vi "Main template.vi"() -> ()   [LabVIEW 2016]
panel:
  out "Finger 5 (little)":dbl(knob) scale=0.0..180.0
  out "Finger 3 (middle)":dbl(knob) scale=0.0..180.0
  out "Finger 4 (ring)":dbl(knob) scale=0.0..180.0
  out "Finger 2 (index)":dbl(knob) scale=0.0..180.0
  out "Finger 1 (thumb)":dbl(knob) scale=0.0..180.0
  out "Finger 5 (individual)":bool
  out "Finger 4 (individual)":bool
  out "Finger 3 (individual)":bool
  out "Finger 2 (individual)":bool
  out "Finger 1 (individual)":bool
  in  "Finger 5 (individual)":bool
  in  "FInger 4 (individual)":bool
  in  "Finger 3 (individual)":bool
  in  "Finger 2 (individual)":bool
  in  "Finger 1 (individual)":bool
  in  "stop":bool
  out "Test 4":bool
  out "Test 3":bool
  out "Test 2":bool
  out "Test 1":bool
  in  "Boolean 2":bool
  in  "Boolean 1":bool
  # "Joakim Nylander Nordström\ncomp3\nNeurotechnology"
  # "Booleans representing the first two\nbits in message from comp2"
  # "Gauge (mätare) displaying\neach finger angle"
  # "Booleans for the last five bits\ncontrolling individual fingers"
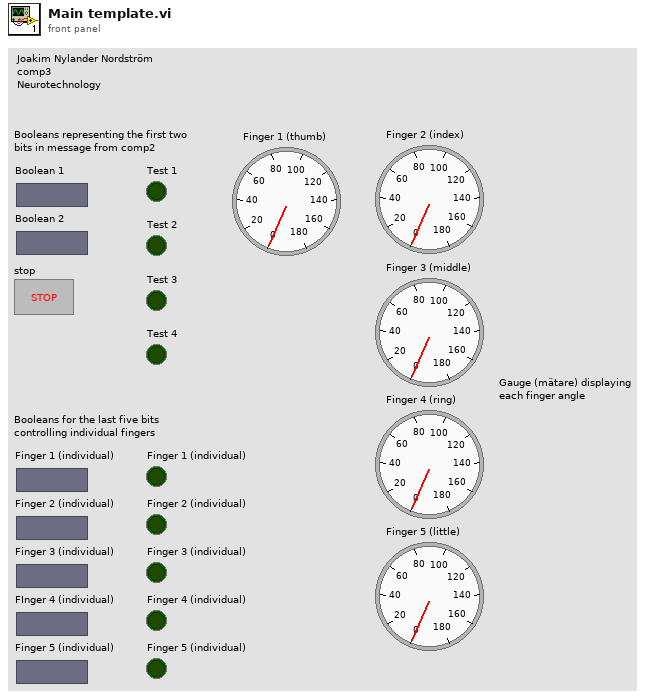
[diagram p1: front panel]
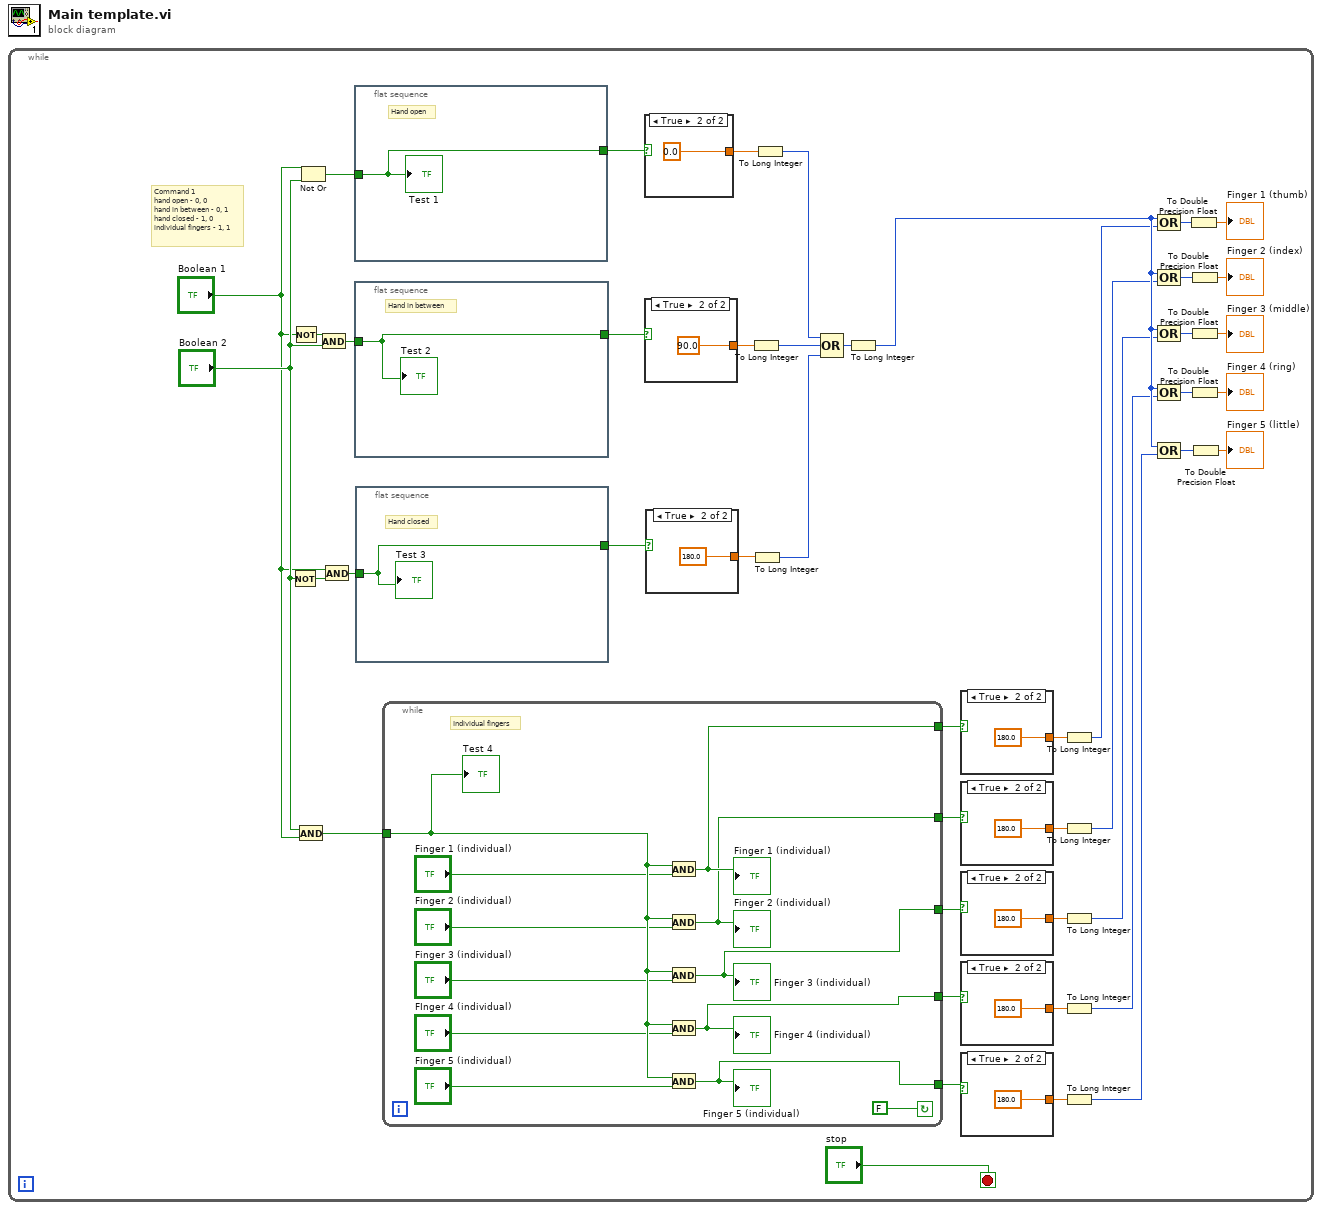
[diagram p0: block diagram]
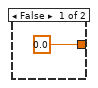
[diagram p2: hidden frame]
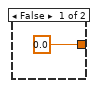
[diagram p3: hidden frame]
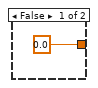
[diagram p4: hidden frame]
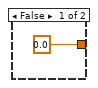
[diagram p5: hidden frame]
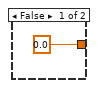
[diagram p6: hidden frame]
diagram:
  n1 = while {
    stop <- "stop" stop-if-true
    # "Command 1\nhand open - 0, 0\nhand in between - 0, 1\nhand closed - 1, 0\nindividual fingers - 1, 1"
    n2 = Not(x="Boolean 2") -> (.not. x?=w44:bool)
    n3 = Not(x="Boolean 1") -> (.not. x?=w45:bool)
    n4 = And(x="Boolean 2", y="Boolean 1") -> (x .and. y?=w43:bool)
    n5 = Not Or(1:"Boolean 2", 2:"Boolean 1") -> (0:w42:bool)
    n6 = And(x=w45, y="Boolean 2") -> (x .and. y?=w41:bool)
    n7 = And(x="Boolean 1", y=w44) -> (x .and. y?=w39:bool)
    n8 = flat-sequence {
      tunnel: w42 -> [w61]
      tunnel: [w61] -> w36
      frame #0 {
        # "Hand open"
        "Test 1" <- w61
      }
    }
    n9 = flat-sequence {
      tunnel: w41 -> [w60]
      tunnel: [w60] -> w38
      frame #0 {
        # "Hand in between"
        "Test 2" <- w60
      }
    }
    n10 = flat-sequence {
      tunnel: w39 -> [w59]
      tunnel: [w59] -> w34
      frame #0 {
        # "Hand closed"
        "Test 3" <- w59
      }
    }
    n11 = while {
      tunnel: w43 -> [w73]
      tunnel: [w66] -> w17
      tunnel: [w65] -> w16
      tunnel: [w64] -> w15
      tunnel: [w63] -> w14
      tunnel: [w62] -> w13
      stop <- FALSE continue-if-true
      # "Individual fingers"
      n12 = And(x=w73, y="Finger 1 (individual)") -> (x .and. y?=w66:bool)
      "Finger 1 (individual)" <- w66
      n13 = And(x=w73, y="Finger 2 (individual)") -> (x .and. y?=w65:bool)
      "Finger 2 (individual)" <- w65
      n14 = And(x=w73, y="Finger 3 (individual)") -> (x .and. y?=w64:bool)
      "Finger 3 (individual)" <- w64
      n15 = And(x=w73, y="FInger 4 (individual)") -> (x .and. y?=w63:bool)
      "Finger 4 (individual)" <- w63
      n16 = And(x=w73, y="Finger 5 (individual)") -> (x .and. y?=w62:bool)
      "Finger 5 (individual)" <- w62
      "Test 4" <- w73
    }
    n17 = case shown="True" w36 {
      tunnel: [_ 0.0] -> w35
      frame False {
      }
      frame True {
      }
    }
    n18 = case shown="True" w38 {
      tunnel: [_ 90.0] -> w37
      frame False {
      }
      frame True {
      }
    }
    n19 = case shown="True" w34 {
      tunnel: [_ 180.0] -> w31
      frame False {
      }
      frame True {
      }
    }
    n20 = To Long Integer(number=w37) -> (32bit integer=w32:i32)
    n21 = To Long Integer(number=w31) -> (32bit integer=w30:i32)
    n22 = To Long Integer(number=w35) -> (32bit integer=w33:i32)
    n23 = Compound Arithmetic op=OR(w33, w32, w30) -> (w29:i32)
    n24 = To Long Integer(number=w29) -> (32bit integer=w28:i32)
    n25 = case shown="True" w17 {
      tunnel: [0.0 180.0] -> w12
      frame False {
      }
      frame True {
      }
    }
    n26 = case shown="True" w16 {
      tunnel: [0.0 180.0] -> w11
      frame False {
      }
      frame True {
      }
    }
    n27 = case shown="True" w15 {
      tunnel: [0.0 180.0] -> w10
      frame False {
      }
      frame True {
      }
    }
    n28 = case shown="True" w14 {
      tunnel: [0.0 180.0] -> w9
      frame False {
      }
      frame True {
      }
    }
    n29 = case shown="True" w13 {
      tunnel: [0.0 180.0] -> w8
      frame False {
      }
      frame True {
      }
    }
    n30 = To Long Integer(number=w12) -> (32bit integer=w7:i32)
    n31 = To Long Integer(number=w11) -> (32bit integer=w6:i32)
    n32 = To Long Integer(number=w10) -> (32bit integer=w5:i32)
    n33 = To Long Integer(number=w9) -> (32bit integer=w4:i32)
    n34 = To Long Integer(number=w8) -> (32bit integer=w3:i32)
    n35 = Compound Arithmetic op=OR(w28, w7) -> (w27:i32)
    n36 = Compound Arithmetic op=OR(w28, w6) -> (w25:i32)
    n37 = Compound Arithmetic op=OR(w28, w5) -> (w23:i32)
    n38 = Compound Arithmetic op=OR(w28, w4) -> (w21:i32)
    n39 = Compound Arithmetic op=OR(w28, w3) -> (w19:i32)
    n40 = To Double Precision Float(number=w27) -> (double precision float=→"Finger 1 (thumb)":dbl)
    n41 = To Double Precision Float(number=w25) -> (double precision float=→"Finger 2 (index)":dbl)
    n42 = To Double Precision Float(number=w23) -> (double precision float=→"Finger 3 (middle)":dbl)
    n43 = To Double Precision Float(number=w21) -> (double precision float=→"Finger 4 (ring)":dbl)
    n44 = To Double Precision Float(number=w19) -> (double precision float=→"Finger 5 (little)":dbl)
  }
